vi "Get Angle.vi"(4 "Axis":T1, 8 "error in (no error)":errorcluster, 11 "instrument.PPMS2 in":refnum<class "instrument.PPMS2.lvclass">) -> (0 "error out":errorcluster, 1 "Status":variant, 2 "Angle (°)":dbl, 3 "instrument.PPMS2 out":refnum<class "instrument.PPMS2.lvclass">)   [LabVIEW 2016, in "instrument.PPMS2.lvclass"]
uses:
  instrument.PPMS2.lvclass
  <userlib>/LevyLab/Levylab Instruments/Instrument Types/Cryostat/Typedefs/Rotator Axis--Enum.ctl
  <userlib>/LevyLab/Levylab Instruments/Instrument Types/Cryostat/Instrument.Cryostat.lvclass
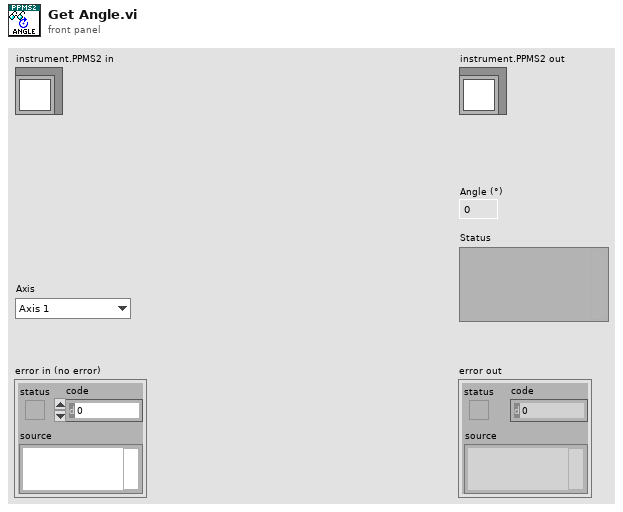
[diagram p1: front panel]
types:
  T1 = typedef "Instrument.Cryostat.lvclass/Rotator Axis--Enum.ctl" = enum16{"Axis 1", "Axis 2"}
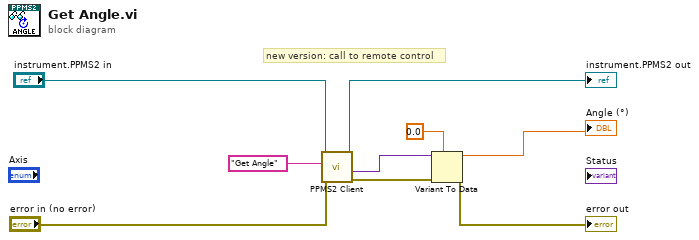
[diagram p0: block diagram]
diagram:
  # "new version: call to remote control"
  n1 = call "PPMS2 Client.vi"("error in (no error)"="error in (no error)", "Command"="Get Angle", "instrument.PPMS2 in"="instrument.PPMS2 in") -> ("error out"=w3:errorcluster, "Data out"=w1:variant, "instrument.PPMS2 out"=→"instrument.PPMS2 out":refnum<class "instrument.PPMS2.lvclass">)  [unwired: 5 in, 1 out]
  n2 = Variant To Data(error in=w3, type=0.0 ("Position (Degree)"), Variant=w1) -> (data=→"Angle (°)":dbl, error out=→"error out":errorcluster)
